vi "Get Grating.vi"(8 "error in (no error)":errorcluster, 11 "Simulated in":refnum<class "Simulated.lvclass">) -> (0 "error out":errorcluster, 2 "Grating ID":u32, 3 "Simulated out":refnum<class "Simulated.lvclass">)   [LabVIEW 2019, in "Simulated.lvclass"]
uses:
  Simulated.lvclass
  Simulated.lvclass/Simulated.ctl
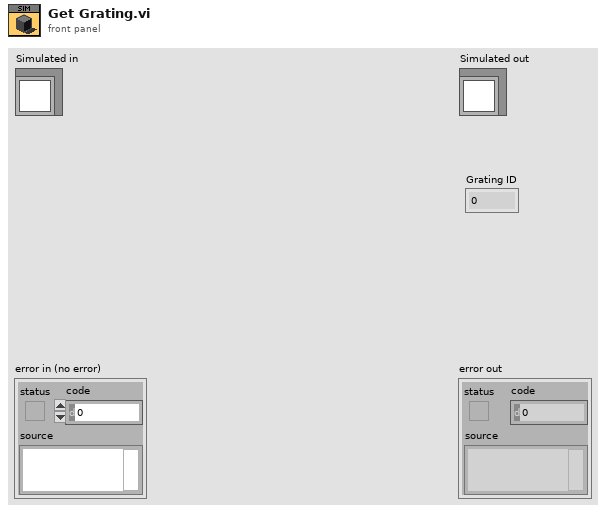
[diagram p1: front panel]
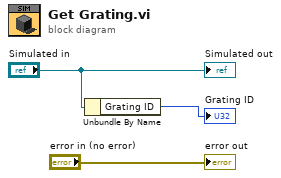
[diagram p0: block diagram]
diagram:
  n1 = Unbundle By Name("Simulated in") -> ("Grating ID"=→"Grating ID":u32)
  "error out" <- "error in (no error)"
  "Simulated out" <- "Simulated in"
